vi "Tosca-Send Timeout.vi"(0 "Time":u32, 7 "State":i32) -> ()   [LabVIEW 2020]
uses:
  Tosca-Message.ctl
  Tosca-Message Action.ctl
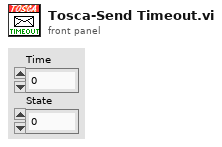
[diagram p1: front panel]
types:
  T1 = typedef "Tosca-Message Action.ctl" = enum16{"None", "Update", "Events", "Timeout", "Error", "Abort"}
  T2 = typedef "Tosca-Message.ctl" = cluster{"Action":T1, "Time":u32, "State":i32, "Events":bool[], "Error":errorcluster}
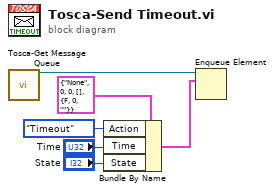
[diagram p0: block diagram]
diagram:
  n1 = call "Tosca-Get Message Queue.vi"() -> ("Message Queue"=w6:refnum<queue>)  [unwired: 14 in, 1 out]
  n2 = Bundle By Name(cluster=T2 {"Action"=enum."None", "Time"=0, "State"=0, "Events"=[], "Error"={"status"=FALSE, "code"=0, "source"=""}} ("element"), "Action"=Tosca-Message_Action."Timeout", "Time"="Time", "State"="State") -> (w3:T2)
  n3 = Enqueue Element(queue=w6, element=w3) -> ()  [unwired: 2 in, 3 out]
